vi "力特性判定.vi"(7 "Result":refnum<vi>, 9 "索引":u8, 10 "判定参数":T1, 11 "XY曲线":cluster{"X":dbl[], "Y":dbl[]}[](array[cluster])) -> (2 "判定项长度":i32, 3 "OK？":bool)   [LabVIEW 2019]
panel:
  out "对称性检测点":dbl
  out "目标5逆向输入扭矩":dbl
  out "目标5正向输入扭矩":dbl
  out "目标 5":dbl
  out "目标4逆向输入扭矩":dbl
  out "目标4正向输入扭矩":dbl
  out "目标 4":dbl
  out "目标3逆向输入扭矩":dbl
  out "目标3正向输入扭矩":dbl
  out "目标 3":dbl
  out "目标2逆向输入扭矩":dbl
  out "目标2正向输入扭矩":dbl
  out "目标 2":dbl
  out "目标1正向输入扭矩":dbl
  out "目标1逆向输入扭矩":dbl
  out "目标 1":dbl
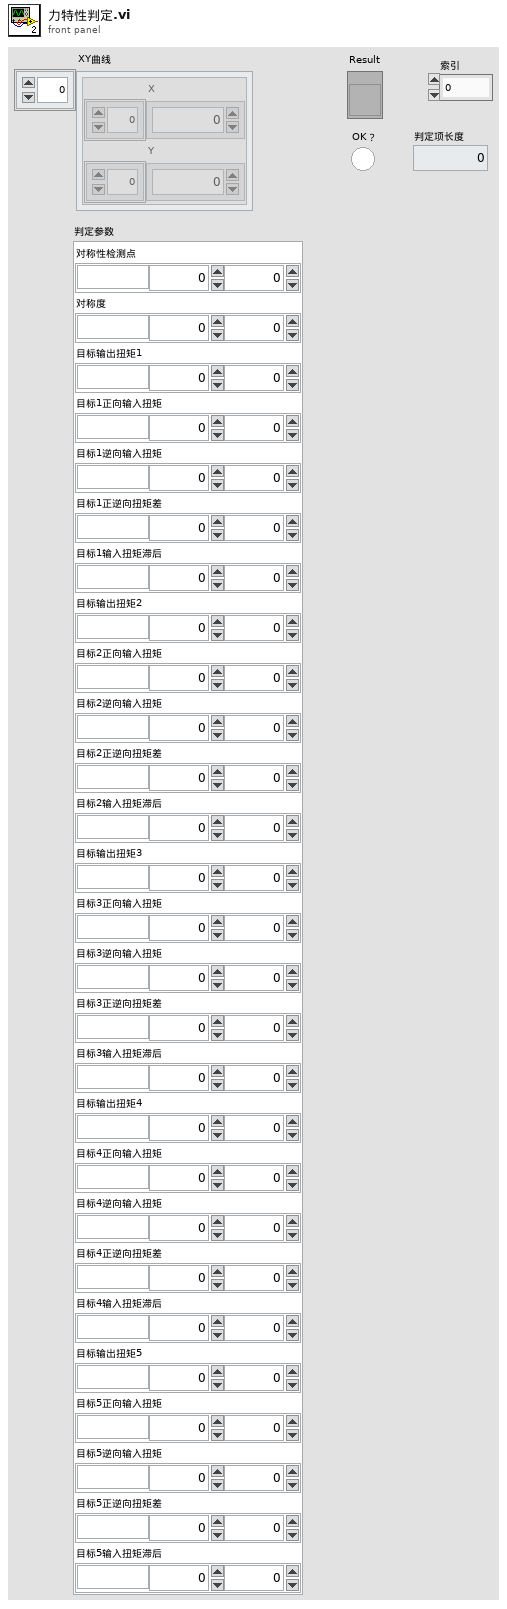
[diagram p1: front panel]
types:
  T1 = cluster{"对称性检测点":cluster{"单位":string, "下限":dbl, "上限":dbl}, "对称度":cluster{"单位":string, "下限":dbl, "上限":dbl}, "目标输出扭矩1":cluster{"单位":string, "下限":dbl, "上限":dbl}, "目标1正向输入扭矩":cluster{"单位":string, "下限":dbl, "上限":dbl}, "目标1逆向输入扭矩":cluster{"单位":string, "下限":dbl, "上限":dbl}, "目标1正逆向扭矩差":cluster{"单位":string, "下限":dbl, "上限":dbl}, "目标1输入扭矩滞后":cluster{"单位":string, "下限":dbl, "上限":dbl}, "目标输出扭矩2":cluster{"单位":string, "下限":dbl, "上限":dbl}, "目标2正向输入扭矩":cluster{"单位":string, "下限":dbl, "上限":dbl}, "目标2逆向输入扭矩":cluster{"单位":string, "下限":dbl, "上限":dbl}, "目标2正逆向扭矩差":cluster{"单位":string, "下限":dbl, "上限":dbl}, "目标2输入扭矩滞后":cluster{"单位":string, "下限":dbl, "上限":dbl}, "目标输出扭矩3":cluster{"单位":string, "下限":dbl, "上限":dbl}, "目标3正向输入扭矩":cluster{"单位":string, "下限":dbl, "上限":dbl}, "目标3逆向输入扭矩":cluster{"单位":string, "下限":dbl, "上限":dbl}, "目标3正逆向扭矩差":cluster{"单位":string, "下限":dbl, "上限":dbl}, "目标3输入扭矩滞后":cluster{"单位":string, "下限":dbl, "上限":dbl}, "目标输出扭矩4":cluster{"单位":string, "下限":dbl, "上限":dbl}, "目标4正向输入扭矩":cluster{"单位":string, "下限":dbl, "上限":dbl}, "目标4逆向输入扭矩":cluster{"单位":string, "下限":dbl, "上限":dbl}, "目标4正逆向扭矩差":cluster{"单位":string, "下限":dbl, "上限":dbl}, "目标4输入扭矩滞后":cluster{"单位":string, "下限":dbl, "上限":dbl}, "目标输出扭矩5":cluster{"单位":string, "下限":dbl, "上限":dbl}, "目标5正向输入扭矩":cluster{"单位":string, "下限":dbl, "上限":dbl}, "目标5逆向输入扭矩":cluster{"单位":string, "下限":dbl, "上限":dbl}, "目标5正逆向扭矩差":cluster{"单位":string, "下限":dbl, "上限":dbl}, "目标5输入扭矩滞后":cluster{"单位":string, "下限":dbl, "上限":dbl}}
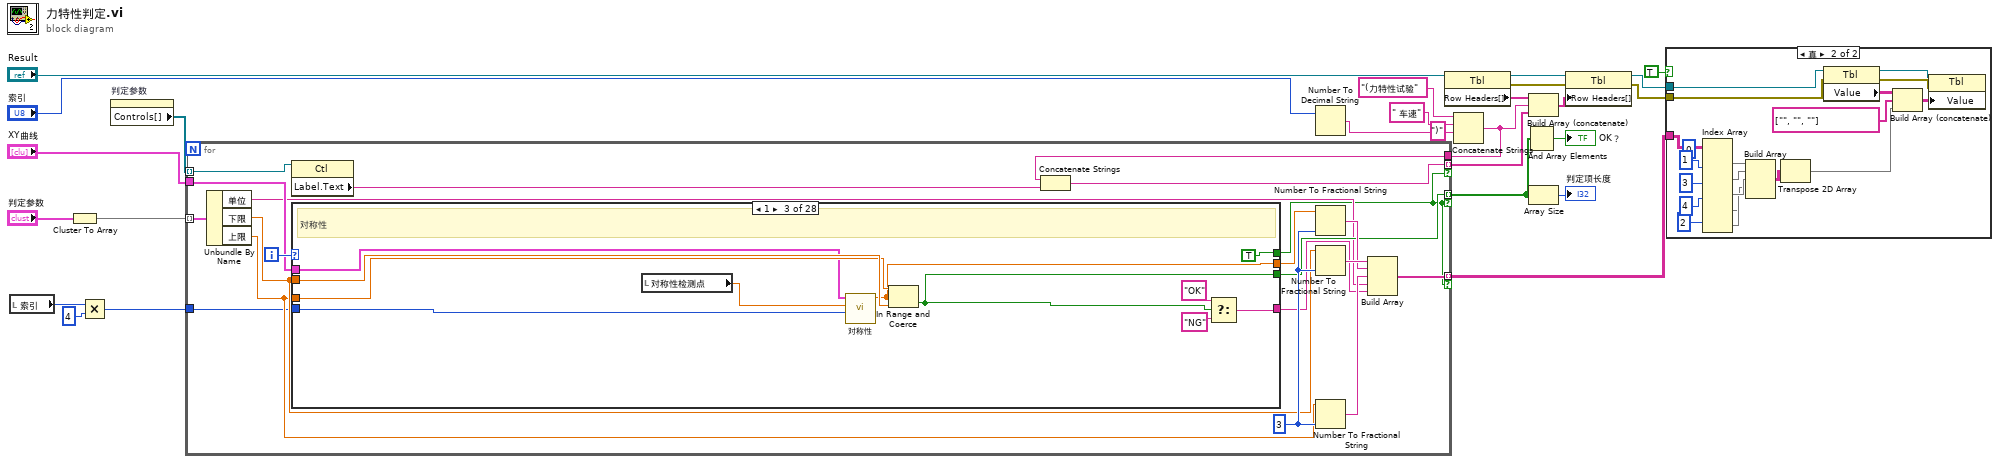
[diagram p0: block diagram]
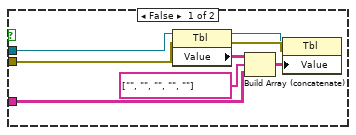
[diagram p2: hidden frame]
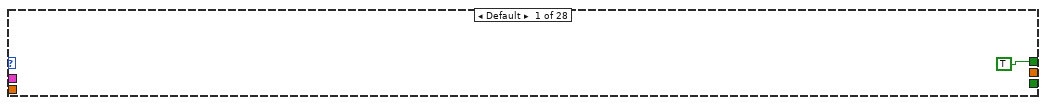
[diagram p3: hidden frame]
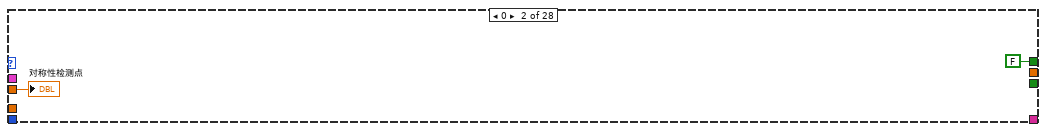
[diagram p4: hidden frame]
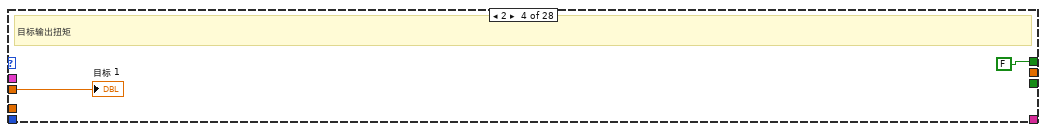
[diagram p5: hidden frame]
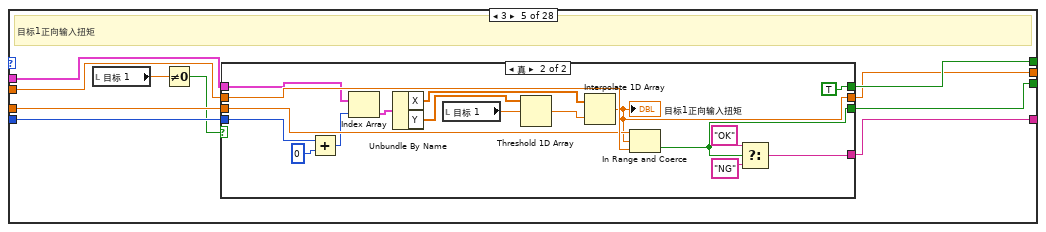
[diagram p6: hidden frame]
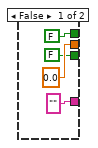
[diagram p7: hidden frame]
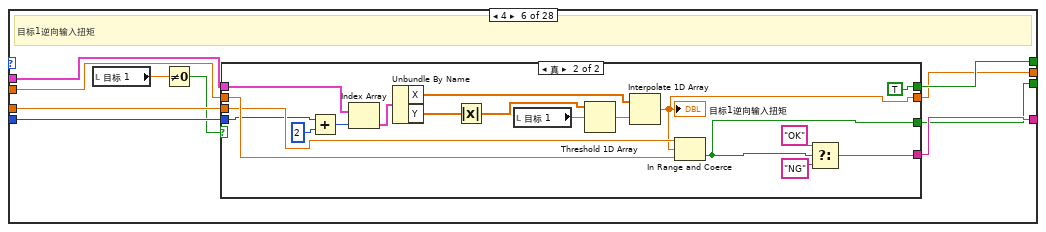
[diagram p8: hidden frame]
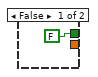
[diagram p9: hidden frame]
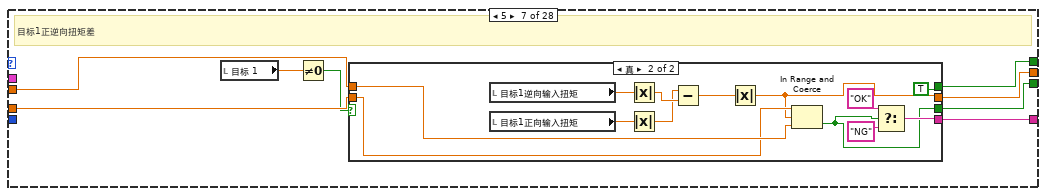
[diagram p10: hidden frame]
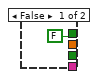
[diagram p11: hidden frame]
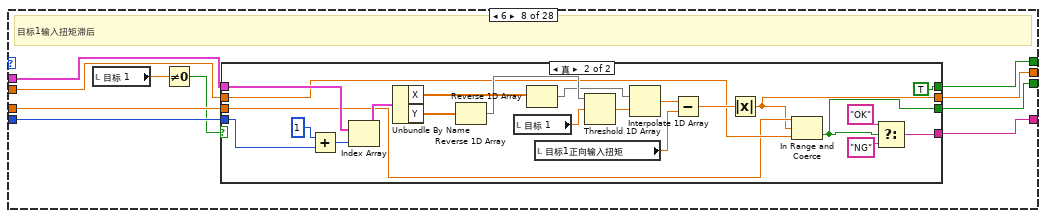
[diagram p12: hidden frame]
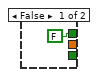
[diagram p13: hidden frame]
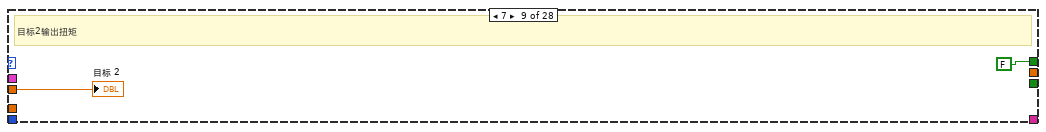
[diagram p14: hidden frame]
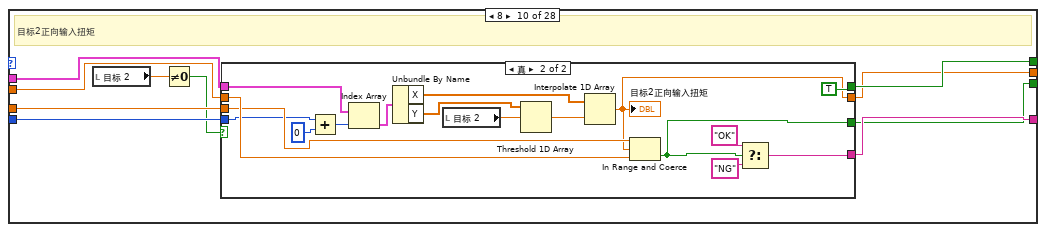
[diagram p15: hidden frame]
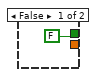
[diagram p16: hidden frame]
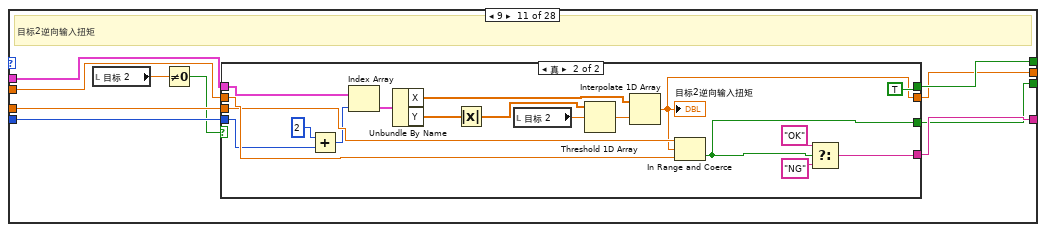
[diagram p17: hidden frame]
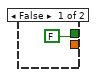
[diagram p18: hidden frame]
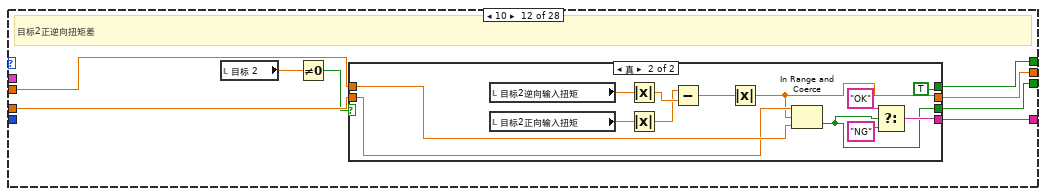
[diagram p19: hidden frame]
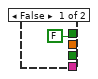
[diagram p20: hidden frame]
diagram:
  n1 = local read "索引"() -> (w7:u8)
  n2 = Cluster To Array(cluster="判定参数") -> (array=w26:cluster{"单位":string, "下限":dbl, "上限":dbl}[])
  n3 = Multiply(x=w7, y=u8 4) -> (x*y=w5:u8)
  n4 = property on="判定参数" class="Clust (严格)"() -> ("Controls[]"=w13:refnum<vi>[])  [unwired: 2 in, 2 out]
  n5 = Number To Decimal String(number="索引") -> (decimal integer string=w10:string)  [unwired: 1 in]
  n6 = property class="Tbl"(reference="Result") -> (reference out=w20:refnum<vi>, error out=w23:errorcluster, "Row Headers[]"=w16:string[])  [unwired: 1 in]
  n7 = Concatenate Strings("(力特性试验" ("Label.Text"), " 车速" ("字符串"), w10, ")" ("字符串")) -> (w1:string)
  n8 = for {
    tunnel: w26 -> [w46] mode=indexing
    tunnel: w13 -> [w44] mode=indexing
    tunnel: "XY曲线" -> [w42]
    tunnel: [w36] -> w4 mode=indexing if=w30
    tunnel: [w32] -> w15 mode=indexing if=w30
    tunnel: [w28] -> w18 mode=indexing if=w30
    tunnel: w5 -> [w29]
    tunnel: w1 -> [w27]
    i -> [w45]
    w41 = i16 3 ("精度(6)")
    n9 = Unbundle By Name(w46) -> ("单位"=w35:string, "下限"=w34:dbl, "上限"=w33:dbl)
    n10 = property class="Ctl"(reference=w44) -> ("Label.Text"=w31:string)  [unwired: 1 in, 2 out]
    n11 = case shown="1" w45 {
      tunnel: [_ _ w52 _ w66 w97 w125 w149 _ w183 w211 w239 w263 _ w297 w325 w353 w377 _ w411 w439 w467 w491 _ w525 w553 w581 w605] -> w43
      tunnel: w42 -> [_ _ w53 _ w67 w98 _ w154 _ w184 w212 _ w268 _ w298 w326 _ w382 _ w412 w440 _ w496 _ w526 w554 _ w610]
      tunnel: [_ _ w58 _ w72 w103 w130 w150 _ w189 w217 w244 w264 _ w303 w331 w358 w378 _ w417 w445 w472 w492 _ w531 w559 w586 w606] -> w37
      tunnel: [_ _ w57 _ w71 w102 w129 w151 _ w188 w216 w243 w265 _ w302 w330 w357 w379 _ w416 w444 w471 w493 _ w530 w558 w585 w607] -> w36
      tunnel: w34 -> [_ w49 w56 w61 w70 w101 w128 w153 w178 w187 w215 w242 w267 w292 w301 w329 w356 w381 w406 w415 w443 w470 w495 w520 w529 w557 w584 w609]
      tunnel: w33 -> [_ _ w55 _ w69 w100 w127 w152 _ w186 w214 w241 w266 _ w300 w328 w355 w380 _ w414 w442 w469 w494 _ w528 w556 w583 w608]
      tunnel: [TRUE FALSE TRUE FALSE w68 w99 w126 w148 FALSE w185 w213 w240 w262 FALSE w299 w327 w354 w376 FALSE w413 w441 w468 w490 FALSE w527 w555 w582 w604] -> w30
      tunnel: w29 -> [_ _ w51 _ w65 w96 _ w147 _ w182 w210 _ w261 _ w296 w324 _ w375 _ w410 w438 _ w489 _ w524 w552 _ w603]
      frame Default {
      }
      frame 0 {
        "对称性检测点" <- w49
      }
      frame 1 {
        # "对称性"
        n12 = local read "对称性检测点"() -> (w50:dbl)
        n13 = call "对称性.vi"("索引"=w51, "定点"=w50, "XY图"=w53) -> ("对称性"=w52:dbl)  [unwired: 8 in]
        n14 = In Range and Coerce(upper limit=w55, x=w52, lower limit=w56) -> (In Range?=w57:bool)  [unwired: 1 out]
        n15 = Select(t="OK", s=w57, f="NG") -> (s? t:f=w58:string)
      }
      frame 2 {
        # "目标输出扭矩"
        "目标 1" <- w61
      }
      frame 3 {
        # "目标1正向输入扭矩"
        n16 = local read "目标 1"() -> (w64:dbl)
        n17 = Not Equal To 0?(x=w64) -> (x != 0?=w63:bool)
        n18 = case shown="真" w63 {
          tunnel: ["" w91] -> w72
          tunnel: [FALSE w90] -> w71
          tunnel: w70 -> [_ w89]
          tunnel: w69 -> [_ w88]
          tunnel: [FALSE TRUE] -> w68
          tunnel: w67 -> [_ w86]
          tunnel: [0.0 w79] -> w66
          tunnel: w65 -> [_ w77]
          frame False {
          }
          frame True {
            n19 = Add(x=w77, y=0 ("索引")) -> (x+y=w78:i32)
            n20 = Index Array(array=w86, index=w78) -> (element=w85:cluster{"X":dbl[], "Y":dbl[]})
            n21 = Unbundle By Name(w85) -> ("X"=w82:dbl[], "Y"=w84:dbl[])
            n22 = local read "目标 1"() -> (w83:dbl)
            n23 = Threshold 1D Array(2:w83, 3:w84) -> (0:w81:dbl)  [unwired: 1 in]
            n24 = Interpolate 1D Array(1:w81, 2:w82) -> (0:w79:dbl)
            "目标1正向输入扭矩" <- w79
            n25 = In Range and Coerce(upper limit=w88, x=w79, lower limit=w89) -> (In Range?=w90:bool)  [unwired: 1 out]
            n26 = Select(t="OK", s=w90, f="NG") -> (s? t:f=w91:string)
          }
        }
      }
      frame 4 {
        # "目标1逆向输入扭矩"
        n27 = local read "目标 1"() -> (w95:dbl)
        n28 = Not Equal To 0?(x=w95) -> (x != 0?=w94:bool)
        n29 = case shown="真" w94 {
          tunnel: [_ w120] -> w103
          tunnel: [_ w119] -> w102
          tunnel: w101 -> [_ w118]
          tunnel: w100 -> [_ w117]
          tunnel: [FALSE TRUE] -> w99
          tunnel: w98 -> [_ w115]
          tunnel: [_ w109] -> w97
          tunnel: w96 -> [_ w105]
          frame False {
          }
          frame True {
            n30 = Add(x=w105, y=2 ("索引")) -> (x+y=w106:i32)
            n31 = Index Array(array=w115, index=w106) -> (element=w114:cluster{"X":dbl[], "Y":dbl[]})
            n32 = Unbundle By Name(w114) -> ("X"=w111:dbl[], "Y"=w113:dbl[])
            n33 = Absolute Value(x=w113) -> (abs(x)=w107:dbl[])
            n34 = local read "目标 1"() -> (w112:dbl)
            n35 = Threshold 1D Array(2:w112, 3:w107) -> (0:w110:dbl)  [unwired: 1 in]
            n36 = Interpolate 1D Array(1:w110, 2:w111) -> (0:w109:dbl)
            "目标1逆向输入扭矩" <- w109
            n37 = In Range and Coerce(upper limit=w117, x=w109, lower limit=w118) -> (In Range?=w119:bool)  [unwired: 1 out]
            n38 = Select(t="OK", s=w119, f="NG") -> (s? t:f=w120:string)
          }
        }
      }
      frame 5 {
        # "目标1正逆向扭矩差"
        n39 = local read "目标 1"() -> (w124:dbl)
        n40 = Not Equal To 0?(x=w124) -> (x != 0?=w123:bool)
        n41 = case shown="真" w123 {
          tunnel: [_ w142] -> w130
          tunnel: [_ w141] -> w129
          tunnel: w128 -> [_ w140]
          tunnel: w127 -> [_ w139]
          tunnel: [FALSE TRUE] -> w126
          tunnel: [_ w134] -> w125
          frame False {
          }
          frame True {
            n42 = local read "目标1逆向输入扭矩"() -> (w136:dbl)
            n43 = local read "目标1正向输入扭矩"() -> (w137:dbl)
            n44 = Absolute Value(x=w136) -> (abs(x)=w133:dbl)
            n45 = Absolute Value(x=w137) -> (abs(x)=w132:dbl)
            n46 = Subtract(x=w132, y=w133) -> (x-y=w135:dbl)
            n47 = Absolute Value(x=w135) -> (abs(x)=w134:dbl)
            n48 = In Range and Coerce(upper limit=w139, x=w134, lower limit=w140) -> (In Range?=w141:bool)  [unwired: 1 out]
            n49 = Select(t="OK", s=w141, f="NG") -> (s? t:f=w142:string)
          }
        }
      }
      frame 6 {
        # "目标1输入扭矩滞后"
        n50 = local read "目标 1"() -> (w146:dbl)
        n51 = Not Equal To 0?(x=w146) -> (x != 0?=w145:bool)
        n52 = case shown="真" w145 {
          tunnel: w154 -> [_ w171]
          tunnel: w153 -> [_ w165]
          tunnel: w152 -> [_ w164]
          tunnel: [_ w161] -> w151
          tunnel: [_ w160] -> w150
          tunnel: [_ w159] -> w149
          tunnel: [FALSE TRUE] -> w148
          tunnel: w147 -> [_ w156]
          frame False {
          }
          frame True {
            n53 = Add(x=1 ("索引"), y=w156) -> (x+y=w157:i32)
            n54 = Index Array(array=w171, index=w157) -> (element=w177:cluster{"X":dbl[], "Y":dbl[]})
            n55 = Unbundle By Name(w177) -> ("X"=w174:dbl[], "Y"=w176:dbl[])
            n56 = Reverse 1D Array(array=w176) -> (reversed array=w170:dbl[])
            n57 = local read "目标 1"() -> (w175:dbl)
            n58 = Reverse 1D Array(array=w174) -> (reversed array=w169:dbl[])
            n59 = local read "目标1正向输入扭矩"() -> (w167:dbl)
            n60 = Threshold 1D Array(2:w175, 3:w170) -> (0:w173:dbl)  [unwired: 1 in]
            n61 = Interpolate 1D Array(1:w173, 2:w169) -> (0:w168:dbl)
            n62 = Subtract(x=w168, y=w167) -> (x-y=w166:dbl)
            n63 = Absolute Value(x=w166) -> (abs(x)=w159:dbl)
            n64 = In Range and Coerce(upper limit=w164, x=w159, lower limit=w165) -> (In Range?=w161:bool)  [unwired: 1 out]
            n65 = Select(t="OK", s=w161, f="NG") -> (s? t:f=w160:string)
          }
        }
      }
      frame 7 {
        # "目标2输出扭矩"
        "目标 2" <- w178
      }
      frame 8 {
        # "目标2正向输入扭矩"
        n66 = local read "目标 2"() -> (w181:dbl)
        n67 = Not Equal To 0?(x=w181) -> (x != 0?=w180:bool)
        n68 = case shown="真" w180 {
          tunnel: [_ w205] -> w189
          tunnel: [_ w204] -> w188
          tunnel: w187 -> [_ w203]
          tunnel: w186 -> [_ w202]
          tunnel: [FALSE TRUE] -> w185
          tunnel: w184 -> [_ w200]
          tunnel: [_ w193] -> w183
          tunnel: w182 -> [_ w191]
          frame False {
          }
          frame True {
            n69 = Add(x=w191, y=0 ("索引")) -> (x+y=w192:i32)
            n70 = Index Array(array=w200, index=w192) -> (element=w199:cluster{"X":dbl[], "Y":dbl[]})
            n71 = Unbundle By Name(w199) -> ("X"=w196:dbl[], "Y"=w198:dbl[])
            n72 = local read "目标 2"() -> (w197:dbl)
            n73 = Threshold 1D Array(2:w197, 3:w198) -> (0:w195:dbl)  [unwired: 1 in]
            n74 = Interpolate 1D Array(1:w195, 2:w196) -> (0:w193:dbl)
            "目标2正向输入扭矩" <- w193
            n75 = In Range and Coerce(upper limit=w202, x=w193, lower limit=w203) -> (In Range?=w204:bool)  [unwired: 1 out]
            n76 = Select(t="OK", s=w204, f="NG") -> (s? t:f=w205:string)
          }
        }
      }
      frame 9 {
        # "目标2逆向输入扭矩"
        n77 = local read "目标 2"() -> (w209:dbl)
        n78 = Not Equal To 0?(x=w209) -> (x != 0?=w208:bool)
        n79 = case shown="真" w208 {
          tunnel: [_ w234] -> w217
          tunnel: [_ w233] -> w216
          tunnel: w215 -> [_ w232]
          tunnel: w214 -> [_ w231]
          tunnel: [FALSE TRUE] -> w213
          tunnel: w212 -> [_ w229]
          tunnel: [_ w223] -> w211
          tunnel: w210 -> [_ w219]
          frame False {
          }
          frame True {
            n80 = Add(x=2 ("索引"), y=w219) -> (x+y=w220:i32)
            n81 = Index Array(array=w229, index=w220) -> (element=w228:cluster{"X":dbl[], "Y":dbl[]})
            n82 = Unbundle By Name(w228) -> ("X"=w225:dbl[], "Y"=w227:dbl[])
            n83 = Absolute Value(x=w227) -> (abs(x)=w221:dbl[])
            n84 = local read "目标 2"() -> (w226:dbl)
            n85 = Threshold 1D Array(2:w226, 3:w221) -> (0:w224:dbl)  [unwired: 1 in]
            n86 = Interpolate 1D Array(1:w224, 2:w225) -> (0:w223:dbl)
            "目标2逆向输入扭矩" <- w223
            n87 = In Range and Coerce(upper limit=w231, x=w223, lower limit=w232) -> (In Range?=w233:bool)  [unwired: 1 out]
            n88 = Select(t="OK", s=w233, f="NG") -> (s? t:f=w234:string)
          }
        }
      }
      frame 10 {
        # "目标2正逆向扭矩差"
        n89 = local read "目标 2"() -> (w238:dbl)
        n90 = Not Equal To 0?(x=w238) -> (x != 0?=w237:bool)
        n91 = case shown="真" w237 {
          tunnel: [_ w256] -> w244
          tunnel: [_ w255] -> w243
          tunnel: w242 -> [_ w254]
          tunnel: w241 -> [_ w253]
          tunnel: [FALSE TRUE] -> w240
          tunnel: [_ w248] -> w239
          frame False {
          }
          frame True {
            n92 = local read "目标2逆向输入扭矩"() -> (w250:dbl)
            n93 = local read "目标2正向输入扭矩"() -> (w251:dbl)
            n94 = Absolute Value(x=w250) -> (abs(x)=w247:dbl)
            n95 = Absolute Value(x=w251) -> (abs(x)=w246:dbl)
            n96 = Subtract(x=w246, y=w247) -> (x-y=w249:dbl)
            n97 = Absolute Value(x=w249) -> (abs(x)=w248:dbl)
            n98 = In Range and Coerce(upper limit=w253, x=w248, lower limit=w254) -> (In Range?=w255:bool)  [unwired: 1 out]
            n99 = Select(t="OK", s=w255, f="NG") -> (s? t:f=w256:string)
          }
        }
      }
      frame 11 {
        # "目标2输入扭矩滞后"
        n100 = local read "目标 2"() -> (w260:dbl)
        n101 = Not Equal To 0?(x=w260) -> (x != 0?=w259:bool)
        n102 = case shown="真" w259 {
          tunnel: w268 -> [_ w285]
          tunnel: w267 -> [_ w279]
          tunnel: w266 -> [_ w278]
          tunnel: [_ w275] -> w265
          tunnel: [_ w274] -> w264
          tunnel: [_ w273] -> w263
          tunnel: [FALSE TRUE] -> w262
          tunnel: w261 -> [_ w270]
          frame False {
          }
          frame True {
            n103 = Add(x=1 ("索引"), y=w270) -> (x+y=w271:i32)
            n104 = Index Array(array=w285, index=w271) -> (element=w291:cluster{"X":dbl[], "Y":dbl[]})
            n105 = Unbundle By Name(w291) -> ("X"=w288:dbl[], "Y"=w290:dbl[])
            n106 = Reverse 1D Array(array=w290) -> (reversed array=w284:dbl[])
            n107 = local read "目标 2"() -> (w289:dbl)
            n108 = Reverse 1D Array(array=w288) -> (reversed array=w283:dbl[])
            n109 = local read "目标2正向输入扭矩"() -> (w281:dbl)
            n110 = Threshold 1D Array(2:w289, 3:w284) -> (0:w287:dbl)  [unwired: 1 in]
            n111 = Interpolate 1D Array(1:w287, 2:w283) -> (0:w282:dbl)
            n112 = Subtract(x=w282, y=w281) -> (x-y=w280:dbl)
            n113 = Absolute Value(x=w280) -> (abs(x)=w273:dbl)
            n114 = In Range and Coerce(upper limit=w278, x=w273, lower limit=w279) -> (In Range?=w275:bool)  [unwired: 1 out]
            n115 = Select(t="OK", s=w275, f="NG") -> (s? t:f=w274:string)
          }
        }
      }
      frame 12 {
        # "目标输出扭矩"
        "目标 3" <- w292
      }
      frame 13 {
        # "目标3正向输入扭矩"
        n116 = local read "目标 3"() -> (w295:dbl)
        n117 = Not Equal To 0?(x=w295) -> (x != 0?=w294:bool)
        n118 = case shown="真" w294 {
          tunnel: [_ w319] -> w303
          tunnel: [_ w318] -> w302
          tunnel: w301 -> [_ w317]
          tunnel: w300 -> [_ w316]
          tunnel: [FALSE TRUE] -> w299
          tunnel: w298 -> [_ w314]
          tunnel: [_ w307] -> w297
          tunnel: w296 -> [_ w305]
          frame False {
          }
          frame True {
            n119 = Add(x=w305, y=0 ("索引")) -> (x+y=w306:i32)
            n120 = Index Array(array=w314, index=w306) -> (element=w313:cluster{"X":dbl[], "Y":dbl[]})
            n121 = Unbundle By Name(w313) -> ("X"=w310:dbl[], "Y"=w312:dbl[])
            n122 = local read "目标 3"() -> (w311:dbl)
            n123 = Threshold 1D Array(2:w311, 3:w312) -> (0:w309:dbl)  [unwired: 1 in]
            n124 = Interpolate 1D Array(1:w309, 2:w310) -> (0:w307:dbl)
            "目标3正向输入扭矩" <- w307
            n125 = In Range and Coerce(upper limit=w316, x=w307, lower limit=w317) -> (In Range?=w318:bool)  [unwired: 1 out]
            n126 = Select(t="OK", s=w318, f="NG") -> (s? t:f=w319:string)
          }
        }
      }
      frame 14 {
        # "目标3逆向输入扭矩"
        n127 = local read "目标 3"() -> (w323:dbl)
        n128 = Not Equal To 0?(x=w323) -> (x != 0?=w322:bool)
        n129 = case shown="真" w322 {
          tunnel: [_ w348] -> w331
          tunnel: [_ w347] -> w330
          tunnel: w329 -> [_ w346]
          tunnel: w328 -> [_ w345]
          tunnel: [FALSE TRUE] -> w327
          tunnel: w326 -> [_ w343]
          tunnel: [_ w337] -> w325
          tunnel: w324 -> [_ w333]
          frame False {
          }
          frame True {
            n130 = Add(x=w333, y=2 ("索引")) -> (x+y=w334:i32)
            n131 = Index Array(array=w343, index=w334) -> (element=w342:cluster{"X":dbl[], "Y":dbl[]})
            n132 = Unbundle By Name(w342) -> ("X"=w339:dbl[], "Y"=w341:dbl[])
            n133 = Absolute Value(x=w341) -> (abs(x)=w335:dbl[])
            n134 = local read "目标 3"() -> (w340:dbl)
            n135 = Threshold 1D Array(2:w340, 3:w335) -> (0:w338:dbl)  [unwired: 1 in]
            n136 = Interpolate 1D Array(1:w338, 2:w339) -> (0:w337:dbl)
            "目标3逆向输入扭矩" <- w337
            n137 = In Range and Coerce(upper limit=w345, x=w337, lower limit=w346) -> (In Range?=w347:bool)  [unwired: 1 out]
            n138 = Select(t="OK", s=w347, f="NG") -> (s? t:f=w348:string)
          }
        }
      }
      frame 15 {
        # "目标3正逆向扭矩差"
        n139 = local read "目标 3"() -> (w352:dbl)
        n140 = Not Equal To 0?(x=w352) -> (x != 0?=w351:bool)
        n141 = case shown="真" w351 {
          tunnel: [_ w370] -> w358
          tunnel: [_ w369] -> w357
          tunnel: w356 -> [_ w368]
          tunnel: w355 -> [_ w367]
          tunnel: [FALSE TRUE] -> w354
          tunnel: [_ w362] -> w353
          frame False {
          }
          frame True {
            n142 = local read "目标3逆向输入扭矩"() -> (w364:dbl)
            n143 = local read "目标3正向输入扭矩"() -> (w365:dbl)
            n144 = Absolute Value(x=w364) -> (abs(x)=w361:dbl)
            n145 = Absolute Value(x=w365) -> (abs(x)=w360:dbl)
            n146 = Subtract(x=w360, y=w361) -> (x-y=w363:dbl)
            n147 = Absolute Value(x=w363) -> (abs(x)=w362:dbl)
            n148 = In Range and Coerce(upper limit=w367, x=w362, lower limit=w368) -> (In Range?=w369:bool)  [unwired: 1 out]
            n149 = Select(t="OK", s=w369, f="NG") -> (s? t:f=w370:string)
          }
        }
      }
      frame 16 {
        # "目标3输入扭矩滞后"
        n150 = local read "目标 3"() -> (w374:dbl)
        n151 = Not Equal To 0?(x=w374) -> (x != 0?=w373:bool)
        n152 = case shown="真" w373 {
          tunnel: w382 -> [_ w399]
          tunnel: w381 -> [_ w393]
          tunnel: w380 -> [_ w392]
          tunnel: [_ w389] -> w379
          tunnel: [_ w388] -> w378
          tunnel: [_ w387] -> w377
          tunnel: [FALSE TRUE] -> w376
          tunnel: w375 -> [_ w384]
          frame False {
          }
          frame True {
            n153 = Add(x=1 ("索引"), y=w384) -> (x+y=w385:i32)
            n154 = Index Array(array=w399, index=w385) -> (element=w405:cluster{"X":dbl[], "Y":dbl[]})
            n155 = Unbundle By Name(w405) -> ("X"=w402:dbl[], "Y"=w404:dbl[])
            n156 = Reverse 1D Array(array=w404) -> (reversed array=w398:dbl[])
            n157 = local read "目标 3"() -> (w403:dbl)
            n158 = Reverse 1D Array(array=w402) -> (reversed array=w397:dbl[])
            n159 = local read "目标3正向输入扭矩"() -> (w395:dbl)
            n160 = Threshold 1D Array(2:w403, 3:w398) -> (0:w401:dbl)  [unwired: 1 in]
            n161 = Interpolate 1D Array(1:w401, 2:w397) -> (0:w396:dbl)
            n162 = Subtract(x=w396, y=w395) -> (x-y=w394:dbl)
            n163 = Absolute Value(x=w394) -> (abs(x)=w387:dbl)
            n164 = In Range and Coerce(upper limit=w392, x=w387, lower limit=w393) -> (In Range?=w389:bool)  [unwired: 1 out]
            n165 = Select(t="OK", s=w389, f="NG") -> (s? t:f=w388:string)
          }
        }
      }
      frame 17 {
        # "目标4输出扭矩"
        "目标 4" <- w406
      }
      frame 18 {
        # "目标4正向输入扭矩"
        n166 = local read "目标 4"() -> (w409:dbl)
        n167 = Not Equal To 0?(x=w409) -> (x != 0?=w408:bool)
        n168 = case shown="真" w408 {
          tunnel: [_ w433] -> w417
          tunnel: [_ w432] -> w416
          tunnel: w415 -> [_ w431]
          tunnel: w414 -> [_ w430]
          tunnel: [FALSE TRUE] -> w413
          tunnel: w412 -> [_ w428]
          tunnel: [_ w421] -> w411
          tunnel: w410 -> [_ w419]
          frame False {
          }
          frame True {
            n169 = Add(x=w419, y=0 ("索引")) -> (x+y=w420:i32)
            n170 = Index Array(array=w428, index=w420) -> (element=w427:cluster{"X":dbl[], "Y":dbl[]})
            n171 = Unbundle By Name(w427) -> ("X"=w424:dbl[], "Y"=w426:dbl[])
            n172 = local read "目标 4"() -> (w425:dbl)
            n173 = Threshold 1D Array(2:w425, 3:w426) -> (0:w423:dbl)  [unwired: 1 in]
            n174 = Interpolate 1D Array(1:w423, 2:w424) -> (0:w421:dbl)
            "目标4正向输入扭矩" <- w421
            n175 = In Range and Coerce(upper limit=w430, x=w421, lower limit=w431) -> (In Range?=w432:bool)  [unwired: 1 out]
            n176 = Select(t="OK", s=w432, f="NG") -> (s? t:f=w433:string)
          }
        }
      }
      frame 19 {
        # "目标4逆向输入扭矩"
        n177 = local read "目标 4"() -> (w437:dbl)
        n178 = Not Equal To 0?(x=w437) -> (x != 0?=w436:bool)
        n179 = case shown="真" w436 {
          tunnel: [_ w462] -> w445
          tunnel: [_ w461] -> w444
          tunnel: w443 -> [_ w460]
          tunnel: w442 -> [_ w459]
          tunnel: [FALSE TRUE] -> w441
          tunnel: w440 -> [_ w457]
          tunnel: [_ w451] -> w439
          tunnel: w438 -> [_ w447]
          frame False {
          }
          frame True {
            n180 = Add(x=w447, y=2 ("索引")) -> (x+y=w448:i32)
            n181 = Index Array(array=w457, index=w448) -> (element=w456:cluster{"X":dbl[], "Y":dbl[]})
            n182 = Unbundle By Name(w456) -> ("X"=w453:dbl[], "Y"=w455:dbl[])
            n183 = Absolute Value(x=w455) -> (abs(x)=w449:dbl[])
            n184 = local read "目标 4"() -> (w454:dbl)
            n185 = Threshold 1D Array(2:w454, 3:w449) -> (0:w452:dbl)  [unwired: 1 in]
            n186 = Interpolate 1D Array(1:w452, 2:w453) -> (0:w451:dbl)
            "目标4逆向输入扭矩" <- w451
            n187 = In Range and Coerce(upper limit=w459, x=w451, lower limit=w460) -> (In Range?=w461:bool)  [unwired: 1 out]
            n188 = Select(t="OK", s=w461, f="NG") -> (s? t:f=w462:string)
          }
        }
      }
      frame 20 {
        # "目标4正逆向扭矩差"
        n189 = local read "目标 4"() -> (w466:dbl)
        n190 = Not Equal To 0?(x=w466) -> (x != 0?=w465:bool)
        n191 = case shown="真" w465 {
          tunnel: [_ w484] -> w472
          tunnel: [_ w483] -> w471
          tunnel: w470 -> [_ w482]
          tunnel: w469 -> [_ w481]
          tunnel: [FALSE TRUE] -> w468
          tunnel: [_ w476] -> w467
          frame False {
          }
          frame True {
            n192 = local read "目标4逆向输入扭矩"() -> (w478:dbl)
            n193 = local read "目标4正向输入扭矩"() -> (w479:dbl)
            n194 = Absolute Value(x=w478) -> (abs(x)=w475:dbl)
            n195 = Absolute Value(x=w479) -> (abs(x)=w474:dbl)
            n196 = Subtract(x=w474, y=w475) -> (x-y=w477:dbl)
            n197 = Absolute Value(x=w477) -> (abs(x)=w476:dbl)
            n198 = In Range and Coerce(upper limit=w481, x=w476, lower limit=w482) -> (In Range?=w483:bool)  [unwired: 1 out]
            n199 = Select(t="OK", s=w483, f="NG") -> (s? t:f=w484:string)
          }
        }
      }
      frame 21 {
        # "目标4输入扭矩滞后"
        n200 = local read "目标 4"() -> (w488:dbl)
        n201 = Not Equal To 0?(x=w488) -> (x != 0?=w487:bool)
        n202 = case shown="真" w487 {
          tunnel: w496 -> [_ w513]
          tunnel: w495 -> [_ w507]
          tunnel: w494 -> [_ w506]
          tunnel: [_ w503] -> w493
          tunnel: [_ w502] -> w492
          tunnel: [_ w501] -> w491
          tunnel: [FALSE TRUE] -> w490
          tunnel: w489 -> [_ w498]
          frame False {
          }
          frame True {
            n203 = Add(x=w498, y=1 ("索引")) -> (x+y=w499:i32)
            n204 = Index Array(array=w513, index=w499) -> (element=w519:cluster{"X":dbl[], "Y":dbl[]})
            n205 = Unbundle By Name(w519) -> ("X"=w516:dbl[], "Y"=w518:dbl[])
            n206 = Reverse 1D Array(array=w518) -> (reversed array=w512:dbl[])
            n207 = local read "目标 4"() -> (w517:dbl)
            n208 = Reverse 1D Array(array=w516) -> (reversed array=w511:dbl[])
            n209 = local read "目标4正向输入扭矩"() -> (w509:dbl)
            n210 = Threshold 1D Array(2:w517, 3:w512) -> (0:w515:dbl)  [unwired: 1 in]
            n211 = Interpolate 1D Array(1:w515, 2:w511) -> (0:w510:dbl)
            n212 = Subtract(x=w510, y=w509) -> (x-y=w508:dbl)
            n213 = Absolute Value(x=w508) -> (abs(x)=w501:dbl)
            n214 = In Range and Coerce(upper limit=w506, x=w501, lower limit=w507) -> (In Range?=w503:bool)  [unwired: 1 out]
            n215 = Select(t="OK", s=w503, f="NG") -> (s? t:f=w502:string)
          }
        }
      }
      frame 22 {
        # "目标5输出扭矩"
        "目标 5" <- w520
      }
      frame 23 {
        # "目标5正向输入扭矩"
        n216 = local read "目标 5"() -> (w523:dbl)
        n217 = Not Equal To 0?(x=w523) -> (x != 0?=w522:bool)
        n218 = case shown="真" w522 {
          tunnel: [_ w547] -> w531
          tunnel: [_ w546] -> w530
          tunnel: w529 -> [_ w545]
          tunnel: w528 -> [_ w544]
          tunnel: [FALSE TRUE] -> w527
          tunnel: w526 -> [_ w542]
          tunnel: [_ w535] -> w525
          tunnel: w524 -> [_ w533]
          frame False {
          }
          frame True {
            n219 = Add(x=0 ("索引"), y=w533) -> (x+y=w534:i32)
            n220 = Index Array(array=w542, index=w534) -> (element=w541:cluster{"X":dbl[], "Y":dbl[]})
            n221 = Unbundle By Name(w541) -> ("X"=w538:dbl[], "Y"=w540:dbl[])
            n222 = local read "目标 5"() -> (w539:dbl)
            n223 = Threshold 1D Array(2:w539, 3:w540) -> (0:w537:dbl)  [unwired: 1 in]
            n224 = Interpolate 1D Array(1:w537, 2:w538) -> (0:w535:dbl)
            "目标5正向输入扭矩" <- w535
            n225 = In Range and Coerce(upper limit=w544, x=w535, lower limit=w545) -> (In Range?=w546:bool)  [unwired: 1 out]
            n226 = Select(t="OK", s=w546, f="NG") -> (s? t:f=w547:string)
          }
        }
      }
      frame 24 {
        # "目标5逆向输入扭矩"
        n227 = local read "目标 5"() -> (w551:dbl)
        n228 = Not Equal To 0?(x=w551) -> (x != 0?=w550:bool)
        n229 = case shown="真" w550 {
          tunnel: [_ w576] -> w559
          tunnel: [_ w575] -> w558
          tunnel: w557 -> [_ w574]
          tunnel: w556 -> [_ w573]
          tunnel: [FALSE TRUE] -> w555
          tunnel: w554 -> [_ w571]
          tunnel: [_ w565] -> w553
          tunnel: w552 -> [_ w561]
          frame False {
          }
          frame True {
            n230 = Add(x=2 ("索引"), y=w561) -> (x+y=w562:i32)
            n231 = Index Array(array=w571, index=w562) -> (element=w570:cluster{"X":dbl[], "Y":dbl[]})
            n232 = Unbundle By Name(w570) -> ("X"=w567:dbl[], "Y"=w569:dbl[])
            n233 = Absolute Value(x=w569) -> (abs(x)=w563:dbl[])
            n234 = local read "目标 5"() -> (w568:dbl)
            n235 = Threshold 1D Array(2:w568, 3:w563) -> (0:w566:dbl)  [unwired: 1 in]
            n236 = Interpolate 1D Array(1:w566, 2:w567) -> (0:w565:dbl)
            "目标5逆向输入扭矩" <- w565
            n237 = In Range and Coerce(upper limit=w573, x=w565, lower limit=w574) -> (In Range?=w575:bool)  [unwired: 1 out]
            n238 = Select(t="OK", s=w575, f="NG") -> (s? t:f=w576:string)
          }
        }
      }
      frame 25 {
        # "目标5正逆向扭矩差"
        n239 = local read "目标 5"() -> (w580:dbl)
        n240 = Not Equal To 0?(x=w580) -> (x != 0?=w579:bool)
        n241 = case shown="真" w579 {
          tunnel: [_ w598] -> w586
          tunnel: [_ w597] -> w585
          tunnel: w584 -> [_ w596]
          tunnel: w583 -> [_ w595]
          tunnel: [FALSE TRUE] -> w582
          tunnel: [_ w590] -> w581
          frame False {
          }
          frame True {
            n242 = local read "目标5逆向输入扭矩"() -> (w592:dbl)
            n243 = local read "目标5正向输入扭矩"() -> (w593:dbl)
            n244 = Absolute Value(x=w592) -> (abs(x)=w589:dbl)
            n245 = Absolute Value(x=w593) -> (abs(x)=w588:dbl)
            n246 = Subtract(x=w588, y=w589) -> (x-y=w591:dbl)
            n247 = Absolute Value(x=w591) -> (abs(x)=w590:dbl)
            n248 = In Range and Coerce(upper limit=w595, x=w590, lower limit=w596) -> (In Range?=w597:bool)  [unwired: 1 out]
            n249 = Select(t="OK", s=w597, f="NG") -> (s? t:f=w598:string)
          }
        }
      }
      frame 26 {
        # "目标5输入扭矩滞后"
        n250 = local read "目标 5"() -> (w602:dbl)
        n251 = Not Equal To 0?(x=w602) -> (x != 0?=w601:bool)
        n252 = case shown="真" w601 {
          tunnel: w610 -> [_ w627]
          tunnel: w609 -> [_ w621]
          tunnel: w608 -> [_ w620]
          tunnel: [_ w617] -> w607
          tunnel: [_ w616] -> w606
          tunnel: [_ w615] -> w605
          tunnel: [FALSE TRUE] -> w604
          tunnel: w603 -> [_ w612]
          frame False {
          }
          frame True {
            n253 = Add(x=1 ("索引"), y=w612) -> (x+y=w613:i32)
            n254 = Index Array(array=w627, index=w613) -> (element=w633:cluster{"X":dbl[], "Y":dbl[]})
            n255 = Unbundle By Name(w633) -> ("X"=w630:dbl[], "Y"=w632:dbl[])
            n256 = Reverse 1D Array(array=w632) -> (reversed array=w626:dbl[])
            n257 = local read "目标 5"() -> (w631:dbl)
            n258 = Reverse 1D Array(array=w630) -> (reversed array=w625:dbl[])
            n259 = local read "目标5正向输入扭矩"() -> (w623:dbl)
            n260 = Threshold 1D Array(2:w631, 3:w626) -> (0:w629:dbl)  [unwired: 1 in]
            n261 = Interpolate 1D Array(1:w629, 2:w625) -> (0:w624:dbl)
            n262 = Subtract(x=w624, y=w623) -> (x-y=w622:dbl)
            n263 = Absolute Value(x=w622) -> (abs(x)=w615:dbl)
            n264 = In Range and Coerce(upper limit=w620, x=w615, lower limit=w621) -> (In Range?=w617:bool)  [unwired: 1 out]
            n265 = Select(t="OK", s=w617, f="NG") -> (s? t:f=w616:string)
          }
        }
      }
    }
    n266 = Concatenate Strings(w27, w31) -> (w28:string)
    n267 = Number To Fractional String(number=w43, precision (6)=w41) -> (F-format string=w39:string)  [unwired: 2 in]
    n268 = Number To Fractional String(number=w34, precision (6)=w41) -> (F-format string=w40:string)  [unwired: 2 in]
    n269 = Number To Fractional String(number=w33, precision (6)=w41) -> (F-format string=w38:string)  [unwired: 2 in]
    n270 = Build Array(w40, w39, w38, w35, w37) -> (w32:string[])
  }
  n271 = And Array Elements(Boolean array=w4) -> (logical AND=→"OK？":bool)
  n272 = Build Array (concatenate)(w16, w1, w18) -> (w19:string[])
  n273 = Array Size(array=w4) -> (size(s)=→"判定项长度":i32)
  n274 = property class="Tbl"(reference=w20, error in=w23, "Row Headers[]"=w19) -> (reference out=w21:refnum<vi>, error out=w22:errorcluster)
  n275 = case shown="真" TRUE {
    tunnel: w22 -> [w639 w659]
    tunnel: w21 -> [w636 w656]
    tunnel: w15 -> [w635 w647]
    frame False {
      n276 = property class="Tbl"(reference=w636, error in=w639) -> (reference out=w637:refnum<vi>, error out=w638:errorcluster, "Value"=w640:string[][])
      n277 = Build Array (concatenate)(w640, string[] ["", "", "", "", ""], w635) -> (w641:string[][])
      n278 = property class="Tbl"(reference=w637, error in=w638, "Value"=w641) -> ()  [unwired: 2 out]
    }
    frame True {
      n279 = Index Array(array=w647, index (col) #1=1 ("禁用的索引 (列)"), index (col) #2=3 ("索引 (列)"), index (col) #3=4 ("索引 (列)"), index (col) #4=0 ("索引 (列)"), index (col) #5=2 ("索引 (列)")) -> (element #1=w651:string[], element #2=w650:string[], element #3=w649:string[], element #4=w642:string[], element #5=w643:string[])  [unwired: 5 in]
      n280 = Build Array(w651, w650, w649, w642, w643) -> (w648:string[][])
      n281 = Transpose 2D Array(2D array=w648) -> (transposed array=w646:string[][])
      n282 = property class="Tbl"(reference=w656, error in=w659) -> (reference out=w657:refnum<vi>, error out=w658:errorcluster, "Value"=w660:string[][])
      n283 = Build Array (concatenate)(w660, string[] ["", "", ""], w646) -> (w661:string[][])
      n284 = property class="Tbl"(reference=w657, error in=w658, "Value"=w661) -> ()  [unwired: 2 out]
    }
  }
